vi "Cast to Child.vi"(8 "error in (no error)":errorcluster, 10 "Parent":refnum<class "Text File.lvclass">, 11 "Child in":refnum<class "Text File.lvclass">) -> (0 "error out":errorcluster, 3 "Child Out":refnum<class "Text File.lvclass">)   [LabVIEW 2019, in "TSC Event Logger.lvlib" / "Text File.lvclass"]
doc: "Pass the parent data down to the child object directly in the casting.\n\n<b>Code Developed By:</b>\nTechnology Service Corporation\nBloomington, IN 47403\nwww.tsc.com/atcs\n\nDeveloper:\nDaniel Coons"
uses:
  Text File.lvclass
  Text File.lvclass/Text File.ctl
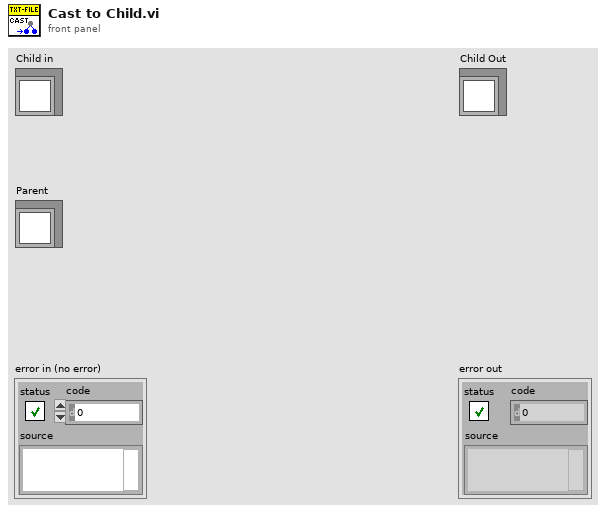
[diagram p1: front panel]
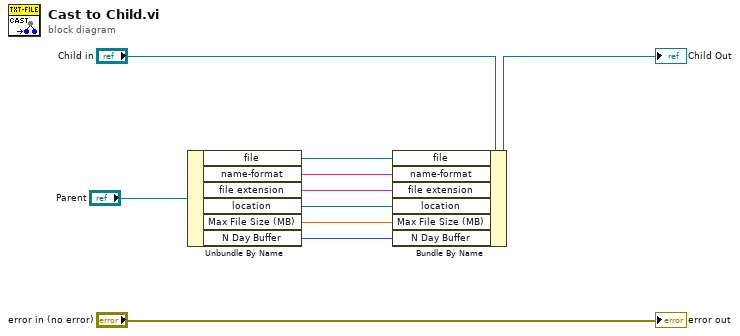
[diagram p0: block diagram]
diagram:
  n1 = Unbundle By Name("Parent") -> ("file"=w6:refnum<file>, "name-format"=w5:string, "file extension"=w4:string, "location"=w3:path, "Max File Size (MB)"=w2:dbl, "N Day Buffer"=w1:u32)
  n2 = Bundle By Name(cluster="Child in", "file"=w6, "name-format"=w5, "file extension"=w4, "location"=w3, "Max File Size (MB)"=w2, "N Day Buffer"=w1) -> (→"Child Out":refnum<class "Text File.lvclass">)
  "error out" <- "error in (no error)"
